vi "SQL-LV Generate Select Function.vi"(8 "error in (no error)":errorcluster, 9 "SQL-LV File Paths.SQL-LV Control Paths":T1, 10 "Table Name":string, 11 "Save as":path) -> (0 "error out":errorcluster, 3 "Save as out":path)   [LabVIEW 2021]
uses:
  SQL-LV Table Control Paths.ctl
  edt.lib/vi_script.lib/Control Replacement Param.ctl
  DB Method Enum.ctl
  edt.lib/vi_script.lib/Constant Replacement Param.ctl
  edt.lib/vi_script.lib/Replace Constant in VI (Scalar).vi
  edt.lib/vi_script.lib/EDT VI Script.lvlib
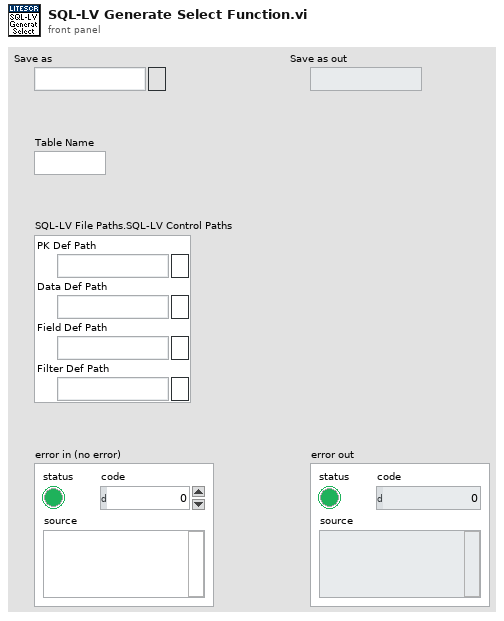
[diagram p1: front panel]
types:
  T1 = typedef "SQL-LV Table Control Paths.ctl" = cluster{"PK Def Path":path, "Data Def Path":path, "Field Def Path":path, "Filter Def Path":path}
  T2 = typedef "EDT VI Script.lvlib/Constant Replacement Param.ctl" = cluster{"Label.Text":string, "Value":variant}
  T3 = typedef "DB Method Enum.ctl" = enum16{"Insert", "Delete", "Select", "Update", "List"}
  T4 = typedef "EDT VI Script.lvlib/Control Replacement Param.ctl" = cluster{"Placeholder Name":string, "CTL File Path":path, "Indicator":bool}
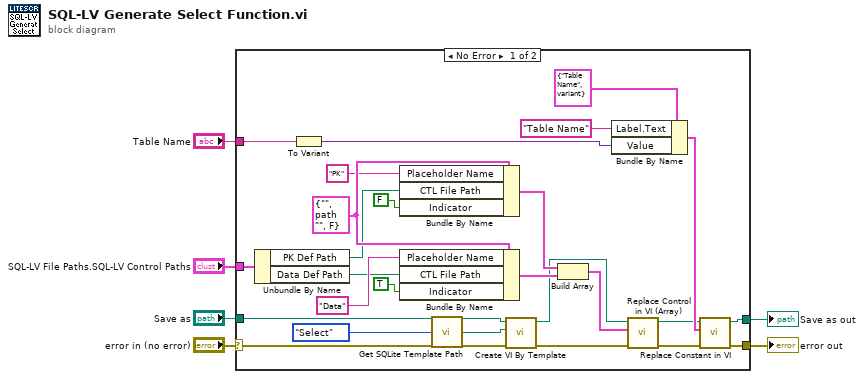
[diagram p0: block diagram]
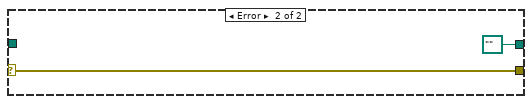
[diagram p2: hidden frame]
diagram:
  n1 = case shown="No Error" "error in (no error)" {
    selector: "error in (no error)" -> [w23 w33]
    tunnel: [w12 path "" ("Save as out")] -> w6
    tunnel: "Save as" -> [w9 _]
    tunnel: [w10 w33] -> w4
    tunnel: "SQL-LV File Paths.SQL-LV Control Paths" -> [w22 _]
    tunnel: "Table Name" -> [w16 _]
    frame No Error {
      w26 = T4 {"Placeholder Name"="", "CTL File Path"=path "", "Indicator"=FALSE} ("Control Replacement Param")
      n2 = Unbundle By Name(w22) -> ("PK Def Path"=w21:path, "Data Def Path"=w20:path)
      n3 = To Variant(anything=w16) -> (Variant=w15:variant)
      n4 = Bundle By Name(cluster=w26, "Placeholder Name"="PK" ("Control Placeholder Name"), "CTL File Path"=w21, "Indicator"=FALSE) -> (w27:T4)
      n5 = Bundle By Name(cluster=w26, "Placeholder Name"="Data" ("Control Placeholder Name"), "CTL File Path"=w20, "Indicator"=TRUE) -> (w28:T4)
      n6 = call "Get SQLite Template Path.vi"("Template Type"=DB_Method_Enum."Select") -> ("Template Path"=w8:path)
      n7 = call "Create VI By Template.vi"("error in"=w23, "Template VI Path"=w8, "Save as"=w9) -> ("error out"=w18:errorcluster, "Save as out"=w19:path)  [unwired: 7 in]
      n8 = Build Array(w27, w28) -> (w31:T4[])
      n9 = Bundle By Name(cluster=T2 {"Label.Text"="Table Name", "Value"=variant} ("Constant Replacement Params"), "Label.Text"="Table Name", "Value"=w15) -> (w14:T2)
      n10 = call "Replace Control in VI (Array).vi"("error in"=w18, "Control Replacement Params"=w31, "Original VI"=w19) -> ("error out"=w11:errorcluster, "Save as out"=w13:path)  [unwired: 7 in]
      n11 = call-poly "Replace Constant in VI.vi"("error in"=w11, "Constant Replacement Params"=w14, "Original VI"=w13) -> ("error out"=w10:errorcluster, "Save as out"=w12:path)  [unwired: 7 in]
    }
    frame Error {
    }
  }
  "Save as out" <- w6
  "error out" <- w4
